vi "getFilePattern.vi"(8 "error in (no error)":errorcluster, 11 "npoiDocument in":refnum<class "npoiDocument.lvclass">) -> (0 "error out":errorcluster, 1 "pattern":string, 2 "pattern label":string, 3 "npoiDocument out":refnum<class "npoiDocument.lvclass">)   [LabVIEW 2017, in "NPOI_Document.lvlib" / "npoiDocument.lvclass"]
uses:
  npoiDocument.lvclass
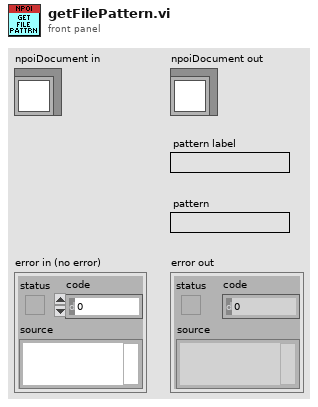
[diagram p1: front panel]
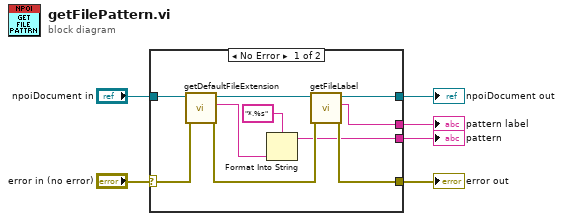
[diagram p0: block diagram]
diagram:
  n1 = case shown="No Error" "error in (no error)" {
    selector: "error in (no error)" -> [w11 w18]
    tunnel: [w9 w18] -> w5
    tunnel: [w13 w17] -> w3
    tunnel: "npoiDocument in" -> [w12 w17]
    tunnel: [w8 _] -> w2
    tunnel: [w7 _] -> w1
    frame No Error {
      n2 = call-dynamic "getDefaultFileExtension.vi"("error in (no error)"=w11, "npoiDocument in"=w12) -> ("error out"=w10:errorcluster, "Default File Extension"=w16:string, "npoiDocument out"=w14:refnum<class "npoiDocument.lvclass">)  [unwired: 7 in]
      n3 = Format Into String(format string="*.%s", w16) -> (resulting string=w7:string)  [unwired: 2 in, 1 out]
      n4 = call-dynamic "getFileLabel.vi"("error in (no error)"=w10, "npoiDocument in"=w14) -> ("error out"=w9:errorcluster, "Default File Label"=w8:string, "npoiDocument out"=w13:refnum<class "npoiDocument.lvclass">)  [unwired: 7 in]
    }
    frame Error {
    }
  }
  "error out" <- w5
  "npoiDocument out" <- w3
  "pattern" <- w1
  "pattern label" <- w2
